vi "idn_action.vi"(0 "HGF_ImaqDx":refnum<class "HGF_ImaqDx.lvclass">, 5 "error in (no error)":errorcluster) -> (12 "resourceString":string, 13 "additionalInfo":string, 14 "HGF_ImaqDx out":refnum<class "HGF_ImaqDx.lvclass">, 15 "driverRevision":string="unknown", 16 "firmwareRevision":string="unknown", 17 "vendor":string="unknown", 18 "model":string="unknown", 19 "error out":errorcluster)   [LabVIEW 2014, in "HGF_IMAQ.lvlib" / "HGF_ImaqDx.lvclass"]
doc: "This VI queries the current instrument firmware revision and instrument driver revision.\n\nFor detailed driver information including modification history, refer to the Readme file.\n\n<b>Hint:</b> This is a dynamic dispatch VI to be implemented by child classes."
uses:
  HGF_ImaqDx.lvclass
  <resource>/objmgr/imaqdx.rc
  HGF_IMAQDevice/HGF_IMAQDevice.lvclass
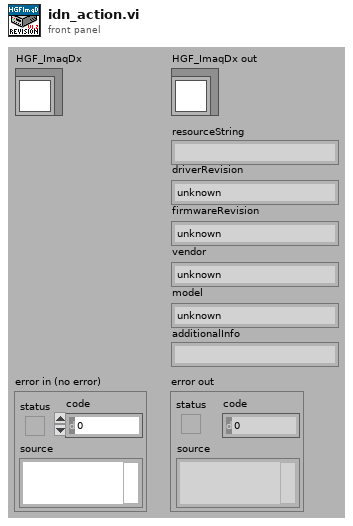
[diagram p1: front panel]
types:
  T1 = typedef "IMAQdx.ctl" = refnum<k21>
  T2 = cluster{"Major":u16, "Minor":u16, "Fix":u16, "Build":u16}
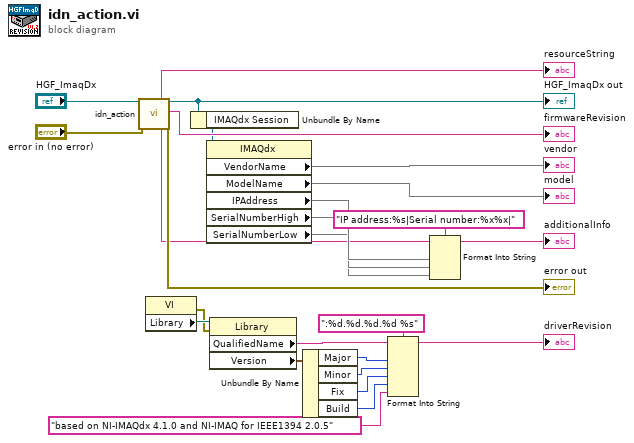
[diagram p0: block diagram]
diagram:
  n1 = call-parent "idn_action.vi"("HGF_IMAQDevice"="HGF_ImaqDx", "error in (no error)"="error in (no error)") -> ("resourceString"=→"resourceString":string, "additionalInfo"=w3:string, "HGF_IMAQDevice out"=w21:refnum<class "HGF_ImaqDx.lvclass">, "firmwareRevision"=→"firmwareRevision":string, "error out"=→"error out":errorcluster)  [unwired: 13 out]
  "HGF_ImaqDx out" <- w21
  n2 = property class="VI"() -> (error out=w11:errorcluster, "Library"=w14:refnum<vi>)  [unwired: 2 in, 1 out]
  n3 = Unbundle By Name(w21) -> ("IMAQdx Session"=w10:T1)
  n4 = property class="IMAQdx"(reference=w10) -> ("VendorName"=→"vendor", "ModelName"=→"model", "IPAddress"=w6, "SerialNumberHigh"=w5, "SerialNumberLow"=w4)  [unwired: 1 in, 2 out]
  n5 = property class="Library"(reference=w14, error in=w11) -> ("QualifiedName"=w12:string, "Version"=w20:T2)  [unwired: 2 out]
  n6 = Unbundle By Name(w20) -> ("Major"=w19:u16, "Minor"=w18:u16, "Fix"=w17:u16, "Build"=w16:u16)
  n7 = Format Into String(format string=":%d.%d.%d.%d %s", initial string=w12, w19, w18, w17, w16, "based on NI-IMAQdx 4.1.0 and NI-IMAQ for IEEE1394 2.0.5" ("driverRevision")) -> (resulting string=→"driverRevision":string)  [unwired: 1 in, 1 out]
  n8 = Format Into String(format string="IP address:%s|Serial number:%x%x|", initial string=w3, w6, w5, w4) -> (resulting string=→"additionalInfo":string)  [unwired: 1 in, 1 out]
